vi "in_one-sided slope.vi"(10 "h[0..1]":dbl[](array[numeric]) format="%_6g", 11 "delta[0..1]":dbl[](array[numeric]) format="%_6g") -> (3 "one-sided slope":dbl format="%_6g")   [LabVIEW 2018, in "NI_Gmath.lvlib"]
uses:
  NI_Gmath.lvlib
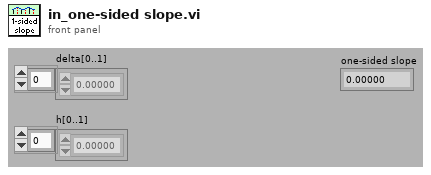
[diagram p1: front panel]
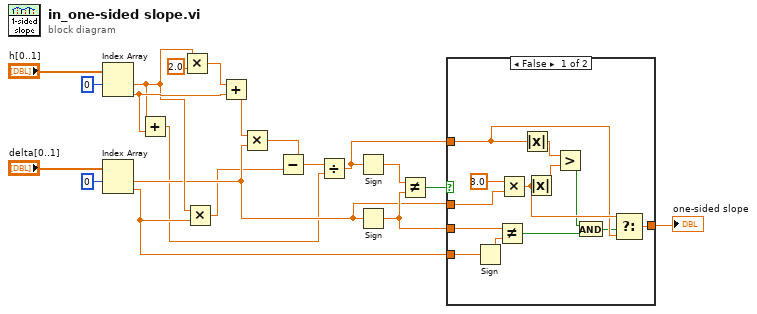
[diagram p0: block diagram]
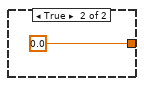
[diagram p2: hidden frame]
diagram:
  n1 = Index Array(array="h[0..1]", index #1=0 ("index")) -> (element #1=w11:dbl, element #2=w12:dbl)  [unwired: 1 in]
  n2 = Index Array(array="delta[0..1]", index #1=0 ("index")) -> (element #1=w6:dbl, element #2=w8:dbl)  [unwired: 1 in]
  n3 = Add(x=w11, y=w12) -> (x+y=w1:dbl)
  n4 = Multiply(x=w11, y=2.0) -> (x*y=w15:dbl)
  n5 = Multiply(x=w11, y=w8) -> (x*y=w4:dbl)
  n6 = Add(x=w15, y=w12) -> (x+y=w14:dbl)
  n7 = Multiply(x=w14, y=w6) -> (x*y=w13:dbl)
  n8 = Subtract(x=w13, y=w4) -> (x-y=w3:dbl)
  n9 = Divide(x=w3, y=w1) -> (x/y=w2:dbl)
  n10 = Sign(1:w2) -> (0:w10:dbl)
  n11 = Sign(1:w6) -> (0:w7:dbl)
  n12 = Not Equal?(x=w10, y=w7) -> (x != y?=w9:bool)
  n13 = case shown="False" w9 {
    tunnel: [w24 0.0] -> w5
    tunnel: w8 -> [w33 _]
    tunnel: w7 -> [w32 _]
    tunnel: w2 -> [w25 _]
    tunnel: w6 -> [w28 _]
    frame False {
      n14 = Sign(1:w33) -> (0:w31:dbl)
      n15 = Not Equal?(x=w32, y=w31) -> (x != y?=w23:bool)
      n16 = Multiply(x=3.0, y=w28) -> (x*y=w26:dbl)
      n17 = Absolute Value(x=w25) -> (abs(x)=w30:dbl)
      n18 = Absolute Value(x=w26) -> (abs(x)=w27:dbl)
      n19 = Greater?(x=w30, y=w27) -> (0:w22:bool)
      n20 = And(x=w22, y=w23) -> (x .and. y?=w21:bool)
      n21 = Select(t=w26, s=w21, f=w25) -> (s? t:f=w24:dbl)
    }
    frame True {
    }
  }
  "one-sided slope" <- w5
